vi "RecorderMainCThread.vi"(5 "Terminate (Boolean CReference)":T1, 7 "NXT":T2={"Hardware"="NXT", "Flattened String"=""}) -> (3 "NXT":T2={"Hardware"="NXT", "Flattened String"=""})   [LabVIEW 2010, in "Packet Recorder.lvlib"]
uses:
  Packet Recorder.lvlib
  <vilib>/NXT/Subs/LVHSConnector.ctl
  CLIB/CRef/Interface/CRef Boolean.llb/Boolean CReference.ctl
  CLIB/CThread/Core/CThread Thread Properties.ctl
  CLIB/CThread/XNodes/referencenode/CThread VI Reference.xnode
  CLIB/CThread/XNodes/terminalnode/CThread VI Terminal Node.xnode
  CLIB/CThread/Base/CThread Base - VI Reference.vi
  CLIB/CThread/Base/CThread Base - While Loop.vi
  CLIB/CRef/Interface/CRef Numeric.llb/I32 CReference.ctl
  CLIB/CRef/CRef.lvlib
  CLIB/CThread/CThread.lvlib
  RecorderMainNoLoop.vi
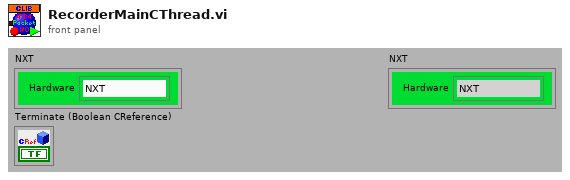
[diagram p1: front panel]
types:
  T1 = typedef "CRef.lvlib/Boolean CReference.ctl" = cluster{"Boolean CRef Address":u16, "Type":enum8{"Null", "Boolean", "U8", "I8", "U16", "I16", "U32", "I32", "U64", "I64", "Single", "Double", "Extended", "CSG", "CDB", "CXT", "Boolean(Def)"}}
  T2 = typedef "LVHSConnector.ctl" = cluster{"Hardware":string, "Flattened String":string}
  T3 = typedef "CThread.lvlib/CThread Thread Properties.ctl" = cluster{"Post-Run Delay (5ms)":u32}
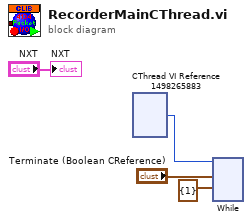
[diagram p0: block diagram]
diagram:
  n1 = xnode "CThread VI Reference 1498265883"() -> ("..\\RecorderMainNoLoop.vi"=w3:i32)
  n2 = xnode "While"("CLIB VI Reference"=w3, "Thread Properties"=T3 {"Post-Run Delay (5ms)"=1}, "CRef: Conditional Terminal"="Terminate (Boolean CReference)") -> ()  [unwired: 2 out]
  "NXT" <- "NXT"
